vi "trash_Benchmark Cleanup.vi"(8 "error in (no error)":errorcluster, 11 "CIFCorePlugin in":refnum<class "CIFCorePlugin.lvclass">) -> (0 "error out":errorcluster, 3 "CIFCorePlugin out":refnum<class "CIFCorePlugin.lvclass">)   [LabVIEW 2021]
uses:
  CIFCorePlugin.lvclass
  CIFCorePlugin.lvclass/CIFCorePlugin.ctl
  Accessors/Timestamps/Read Cleanup TS.vi
  Accessors/Get Time.vi
  CIFUtilities/CIFClocks/SubVIs/Add Error.vi
  CIFUtilities/CIFClocks/Core/Get Time.vi
  Accessors/Read ClockID.vi
  CIFUtilities/CIFClocks/Time Conversion/LabVIEW Time to UTC Time.vi
  CIFCoreCommon/CIFCoreCommon.lvlib
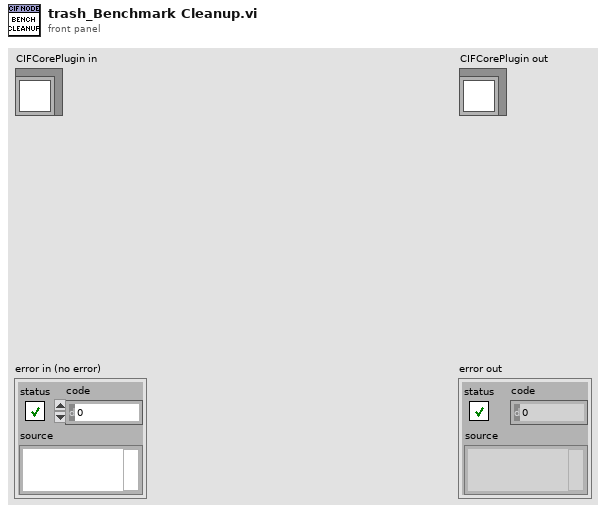
[diagram p1: front panel]
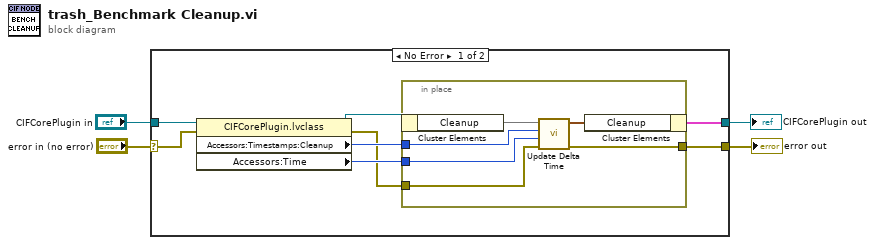
[diagram p0: block diagram]
diagram:
  n1 = case shown="No Error" "error in (no error)" {
    selector: "error in (no error)" -> [w9 w20]
    tunnel: [w12 w20] -> w1
    tunnel: [w7 w19] -> w2
    tunnel: "CIFCorePlugin in" -> [w11 w19]
    frame No Error {
      n2 = property class="CIFCorePlugin.lvclass"(reference=w11, error in=w9) -> (reference out=w8:refnum<class "CIFCorePlugin.lvclass">, error out=w5:errorcluster, "Accessors:Timestamps:Cleanup"=w10:u64, "Accessors:Time"=w6:u64)
      n3 = in-place {
        in-place-border: w5 -> [w18]
        in-place-border: w6 -> [w17]
        in-place-border: [w16] -> w12
        in-place-border: w10 -> [w15]
        n4 = in-place-cluster #1(w8) -> ("Cleanup"=w14)
        n5 = call "Update Delta Time.vi"("error in (no error)"=w18, "T2"=w17, "T1"=w15, "Timing in"=w14) -> ("error out"=w16:errorcluster, "Timing out"=w13:cluster{"Max":i32, "Min":i32})  [unwired: 6 in]
        n6 = in-place-cluster #1("Cleanup"=w13) -> (w7:cluster{})
      }
    }
    frame Error {
    }
  }
  "error out" <- w1
  "CIFCorePlugin out" <- w2
